vi "display.vi"(0 "data":T1[](array[typedef]) {"time (global)" format="%<%H:%M:%S\n%d/%m/%Y>T"}, 5 "raw data buffer":string[](array[string]), 7 "measurement data":dbl[][](array[numeric]), 9 "buffer plot":cluster{"X":dbl[], "Y":dbl[]}) -> (6 "raw data buffer out":string[](array[string]), 10 "buffer plot out":cluster{"X":dbl[], "Y":dbl[]})   [LabVIEW 2010, in "Licor-Steuerung.lvlib"]
uses:
  Licor-Steuerung.lvlib
  LicorLI7000/conventions/output line.ctl
  util/util.lvlib
  LicorLI7000/LicorLI7000.lvlib
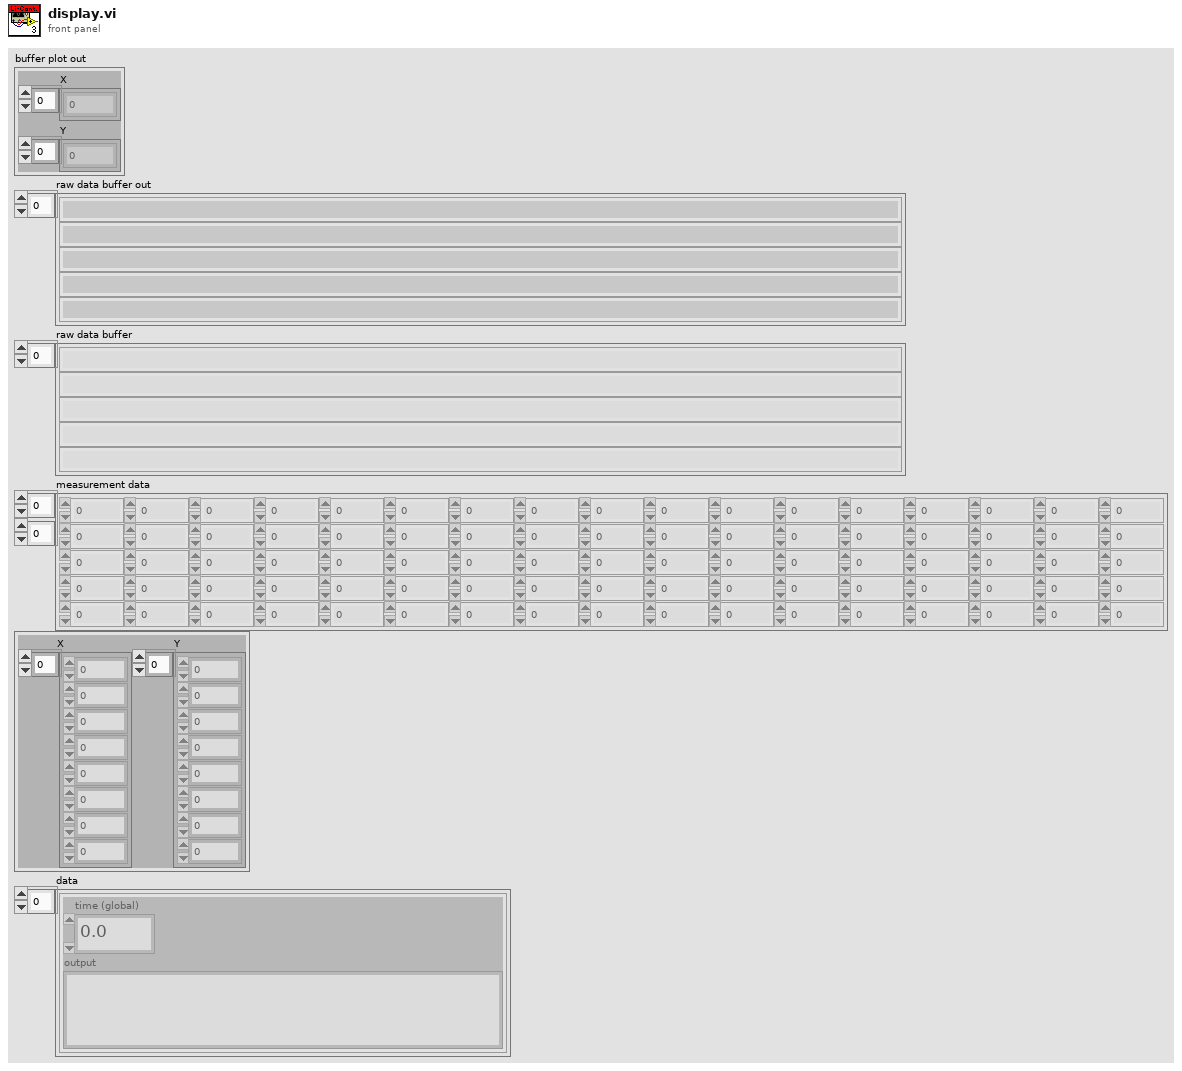
[diagram p1: front panel]
types:
  T1 = typedef "LicorLI7000.lvlib/output line.ctl" = cluster{"time (global)":dbl, "output":string}
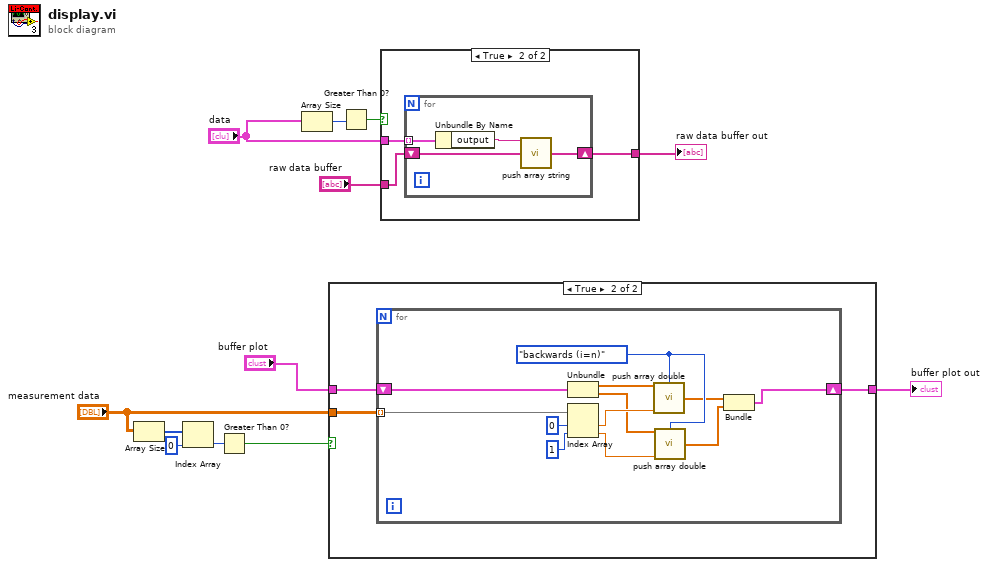
[diagram p0: block diagram]
diagram:
  n1 = Array Size(array="measurement data") -> (size(s)=w7:i32[])
  n2 = Index Array(array=w7, index=0 ("Index")) -> (element=w5:i32)
  n3 = Greater Than 0?(x=w5) -> (x > 0?=w2:bool)
  n4 = Array Size(array="data") -> (size(s)=w11:i32)
  n5 = case shown="True" w2 {
    tunnel: "measurement data" -> [_ w16]
    tunnel: "buffer plot" -> [w13 w15]
    tunnel: [w13 w14] -> w3
    frame False {
    }
    frame True {
      n6 = for {
        tunnel: w16 -> [w28] mode=indexing
        shift-right: [w27] -> w14
        shift-left: w15 -> [w26]
        w19 = enum16{"forwards (i=0)", "backwards (i=n)"}."backwards (i=n)" ("mode")
        n7 = Unbundle(w26) -> ("X"=w22:dbl[], "Y"=w21:dbl[])
        n8 = Index Array(array=w28, index #1=0 ("Index"), index #2=1 ("Index")) -> (element #1=w25:dbl, element #2=w20:dbl)
        n9 = call "push array double.vi"("Array"=w22, "mode"=w19, "Element"=w25) -> ("Array out"=w18:dbl[])  [unwired: 12 in]
        n10 = call "push array double.vi"("Array"=w21, "mode"=w19, "Element"=w20) -> ("Array out"=w17:dbl[])  [unwired: 12 in]
        n11 = Bundle("Array out"=w18, "Array out"=w17) -> (w27:cluster{"Array out":dbl[], "Array out":dbl[]})  [unwired: 1 in]
      }
    }
  }
  "buffer plot out" <- w3
  n12 = Greater Than 0?(x=w11) -> (x > 0?=w10:bool)
  n13 = case shown="True" w10 {
    tunnel: "data" -> [_ w30]
    tunnel: [w29 w32] -> w8
    tunnel: "raw data buffer" -> [w29 w31]
    frame False {
    }
    frame True {
      n14 = for {
        shift-right: [w36] -> w32
        shift-left: w31 -> [w35]
        tunnel: w30 -> [w34] mode=indexing
        n15 = Unbundle By Name(w34) -> ("output"=w33:string)
        n16 = call "push array string.vi"("Element"=w33, "Array"=w35) -> ("Array out"=w36:string[])  [unwired: 13 in]
      }
    }
  }
  "raw data buffer out" <- w8
